vi "PIM Format IM for Plot.vi"(4 "IM Units (\"dBm\" or \"dBc\")":string="dBm", 5 "Measured PIM, dBm":dbl[](array[numeric]) format="%.2f", 6 "Offsets, dB or X":dbl[](array[numeric]) format="%.2f", 7 "RF On/Off":bool[](array[boolean]), 8 "Measured Power, dBm":dbl[](array[numeric]) format="%.2f") -> (0 "Measured PIM, dBm or dBc":dbl[](array[numeric]) format="%.2f")   [LabVIEW 2011]
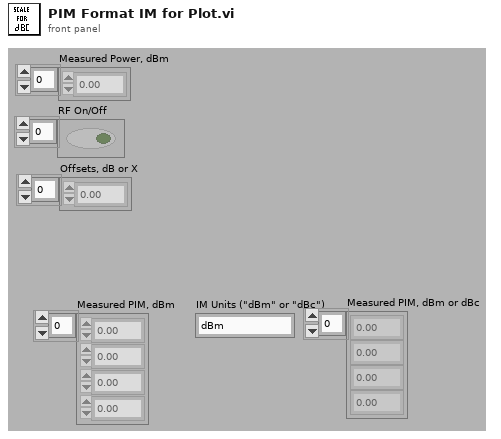
[diagram p1: front panel]
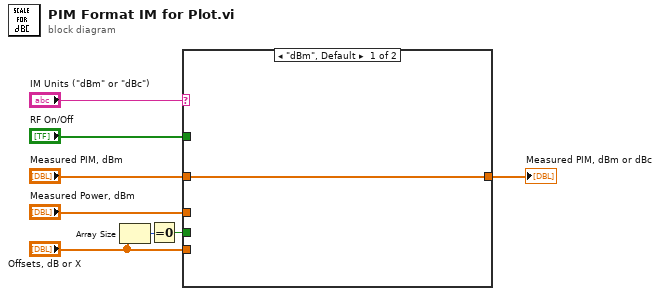
[diagram p0: block diagram]
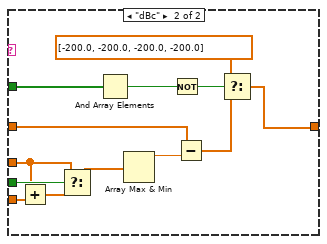
[diagram p2: hidden frame]
diagram:
  n1 = Array Size(array="Offsets, dB or X") -> (size(s)=w2:i32)
  n2 = Equal To 0?(x=w2) -> (x = 0?=w1:bool)
  n3 = case shown="\"dBm\", Default" "IM Units (\"dBm\" or \"dBc\")" {
    tunnel: "Measured PIM, dBm" -> [w9 w22]
    tunnel: [w9 w18] -> w8
    tunnel: "RF On/Off" -> [_ w21]
    tunnel: "Measured Power, dBm" -> [_ w12]
    tunnel: "Offsets, dB or X" -> [_ w15]
    tunnel: w1 -> [_ w13]
    frame "dBm", Default {
    }
    frame "dBc" {
      n4 = Add(x=w12, y=w15) -> (x+y=w11:dbl[])
      n5 = Select(t=w12, s=w13, f=w11) -> (s? t:f=w10:dbl[])
      n6 = And Array Elements(Boolean array=w21) -> (logical AND=w20:bool)
      n7 = Array Max & Min(array=w10) -> (max value=w16:dbl)  [unwired: 3 out]
      n8 = Not(x=w20) -> (.not. x?=w17:bool)
      n9 = Subtract(x=w22, y=w16) -> (x-y=w19:dbl[])
      n10 = Select(t=dbl[] [-200.0, -200.0, -200.0, -200.0] ("initialized array"), s=w17, f=w19) -> (s? t:f=w18:dbl[])
    }
  }
  "Measured PIM, dBm or dBc" <- w8
